vi "Werte ändern (DBL_0xZ.I._Rampen) (SubVI).vi"(0 "geladene Werte (Zeit (s); Wert)":dbl[][](array[numeric]), 1 "Zykluslänge":dbl, 3 "Info":string) -> (5 "Ausgang":dbl[][](array[numeric]) format="%.2f", 6 "Sperre":bool)   [LabVIEW 2010]
panel:
  out "abkühlen C°/s":dbl[](array[numeric])
  in  "abkühlen C°/s":dbl[](array[numeric])
  in  "Zykluslänge 2":dbl
  in  "abkühlen":dbl[](array[numeric])
  in  "Temp warm":dbl[](array[numeric])
  in  "°C/s":dbl[](array[numeric]) format="%#_1f"
  in  "Rampe los":dbl[](array[numeric])
  in  "Temp kalt":dbl[](array[numeric])
  out "abkühlen [s]":dbl[](array[numeric])
  out "Temp warm [°C ]":dbl[](array[numeric])
  out "°C/s":dbl[](array[numeric])
  out "Temp kalt [°C ]":dbl[](array[numeric])
  out "Rampe los [s]":dbl[](array[numeric])
  out "Fehlermeldung":string="Zeit ist größer als Zykluslänge"
  in  "löschen":bool
  out "XY Graph":cluster{"Array":dbl[], "Temp kalt":dbl[]}[](graph) caption="XY-Graph"
  out "Zykluslänge":dbl format="%.2f"
  out "Info":string
  in  "ändern":bool
  in  "Stopp":bool
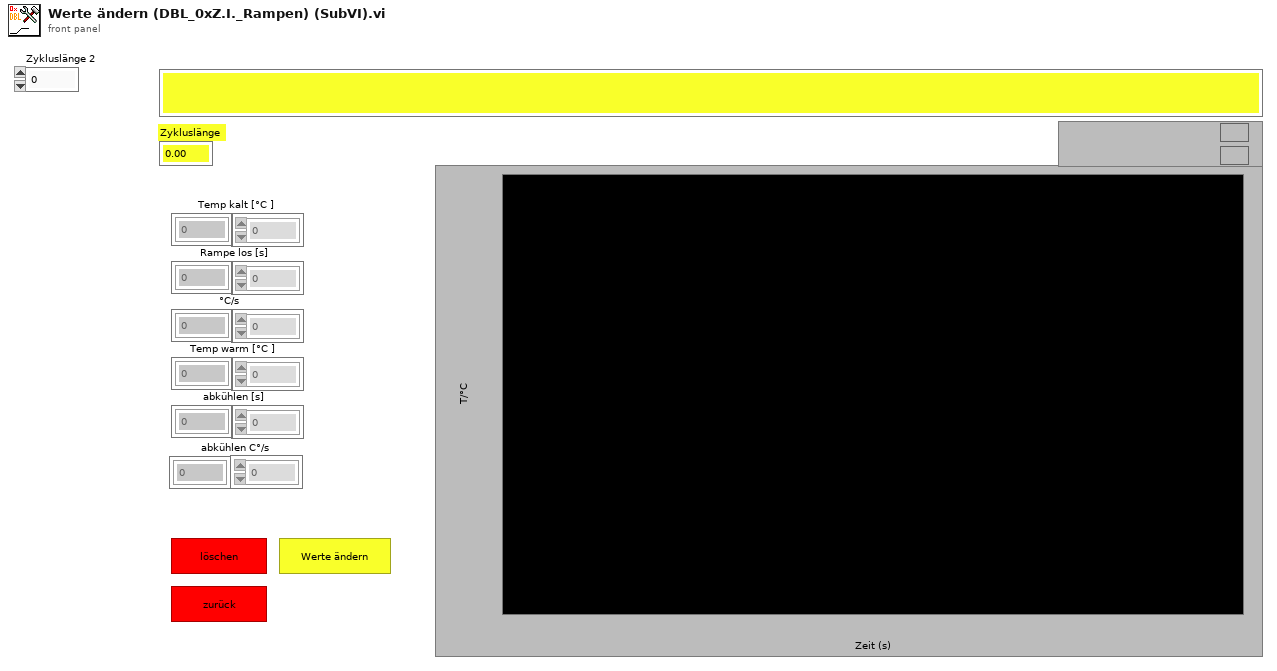
[diagram p1: front panel]
types:
  T1 = cluster{"Array":dbl[], "geladene Werte (Zeit (s); Wert)":dbl[]}
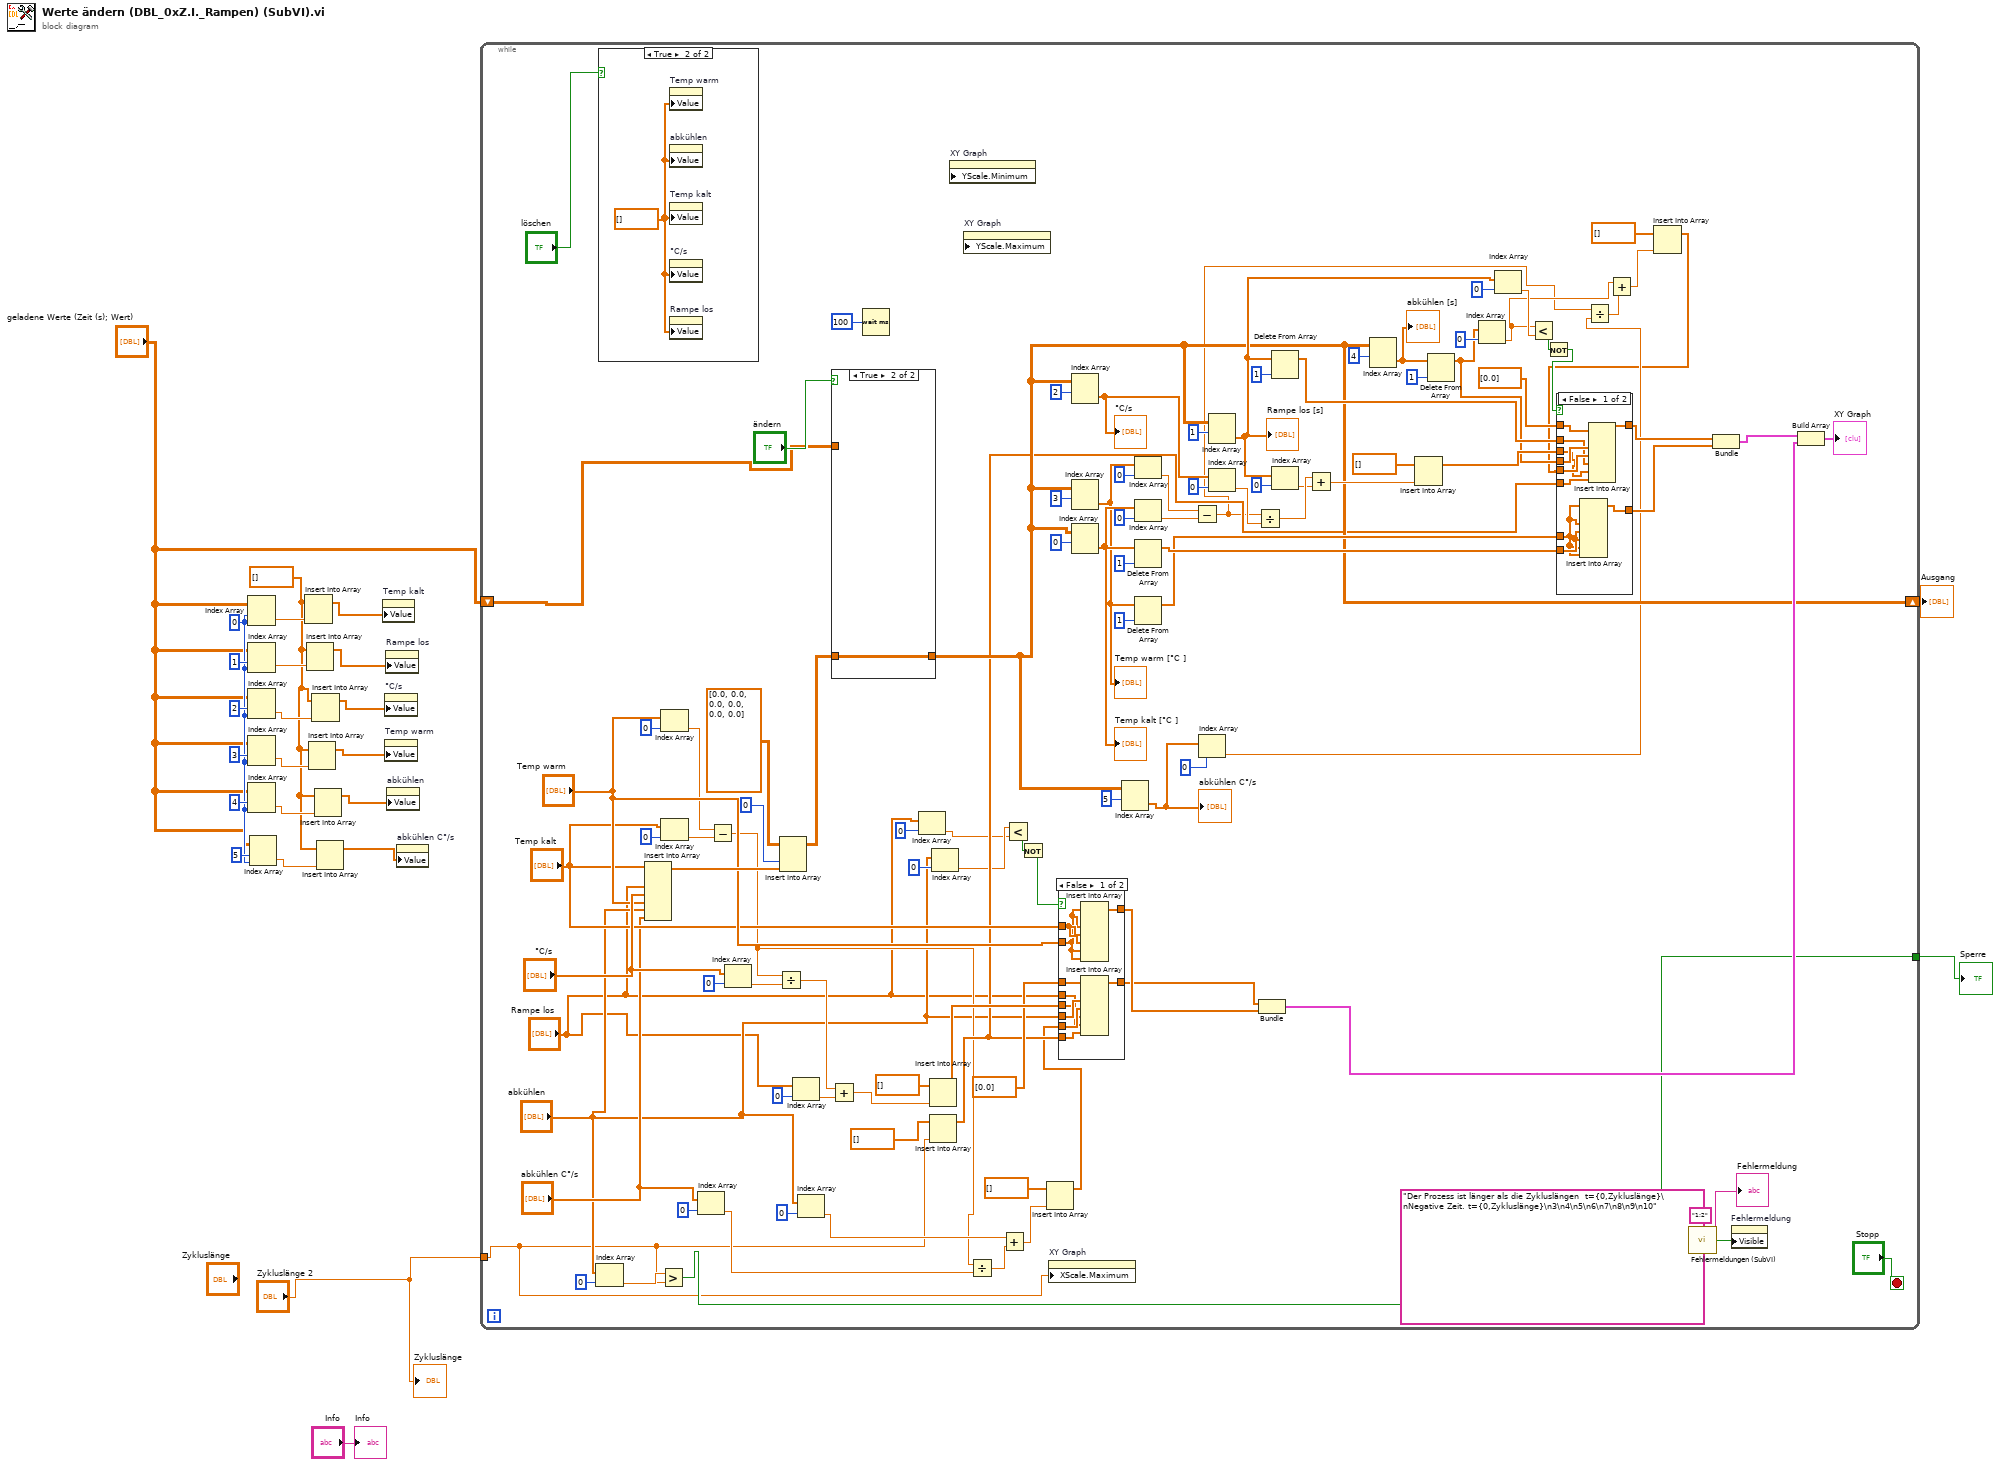
[diagram p0: block diagram]
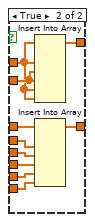
[diagram p2: hidden frame]
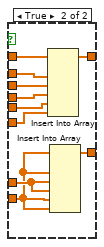
[diagram p3: hidden frame]
diagram:
  w2 = dbl[] [] ("Array")
  w4 = 0 ("Deaktivierter Index (Spalte)")
  n1 = Index Array(array="geladene Werte (Zeit (s); Wert)", index (row)=w4, index (col)=w4) -> (element=w18:dbl)
  n2 = Index Array(array="geladene Werte (Zeit (s); Wert)", index (row)=1 ("Deaktivierter Index (Zeile)"), index (col)=w4) -> (element=w17:dbl)
  n3 = Index Array(array="geladene Werte (Zeit (s); Wert)", index (row)=2 ("Deaktivierter Index (Zeile)"), index (col)=w4) -> (element=w16:dbl)
  n4 = Index Array(array="geladene Werte (Zeit (s); Wert)", index (row)=3 ("Deaktivierter Index (Zeile)"), index (col)=w4) -> (element=w15:dbl)
  n5 = Index Array(array="geladene Werte (Zeit (s); Wert)", index (row)=4 ("Deaktivierter Index (Zeile)"), index (col)=w4) -> (element=w14:dbl)
  n6 = Index Array(array="geladene Werte (Zeit (s); Wert)", index (row)=5 ("Deaktivierter Index (Zeile)"), index (col)=w4) -> (element=w5:dbl)
  n7 = Insert Into Array(array=w2, new element=w18) -> (w10:dbl[])  [unwired: 1 in]
  n8 = Insert Into Array(array=w2, new element=w17) -> (w13:dbl[])  [unwired: 1 in]
  n9 = Insert Into Array(array=w2, new element=w15) -> (w9:dbl[])  [unwired: 1 in]
  n10 = Insert Into Array(array=w2, new element=w16) -> (w12:dbl[])  [unwired: 1 in]
  n11 = Insert Into Array(array=w2, new element=w14) -> (w11:dbl[])  [unwired: 1 in]
  n12 = Insert Into Array(array=w2, new element=w5) -> (w1:dbl[])  [unwired: 1 in]
  n13 = property on="Temp kalt" class="Arr (strikt)"("Value"=w10) -> ()  [unwired: 2 in, 2 out]
  n14 = property on="°C/s" class="Arr (strikt)"("Value"=w12) -> ()  [unwired: 2 in, 2 out]
  n15 = property on="Temp warm" class="Arr (strikt)"("Value"=w9) -> ()  [unwired: 2 in, 2 out]
  n16 = property on="Rampe los" class="Arr (strikt)"("Value"=w13) -> ()  [unwired: 2 in, 2 out]
  n17 = property on="abkühlen" class="Arr (strikt)"("Value"=w11) -> ()  [unwired: 2 in, 2 out]
  n18 = property on="abkühlen C°/s" class="Arr (strikt)"("Value"=w1) -> ()  [unwired: 2 in, 2 out]
  n19 = while {
    shift-right: [w56] -> w24
    shift-left: "geladene Werte (Zeit (s); Wert)" -> [w73]
    tunnel: "Zykluslänge 2" -> [w25]
    tunnel: [w65] -> w8
    stop <- "Stopp" stop-if-true
    n20 = Index Array(array="abkühlen", index=0 ("Index")) -> (element=w71:dbl)
    n21 = case shown="True" "löschen" {
      frame False {
      }
      frame True {
        w173 = dbl[] [] ("neue Werte (Zeit (s); Wert)")
        n22 = property on="Temp warm" class="Arr (strikt)"("Value"=w173) -> ()  [unwired: 2 in, 2 out]
        n23 = property on="abkühlen" class="Arr (strikt)"("Value"=w173) -> ()  [unwired: 2 in, 2 out]
        n24 = property on="Temp kalt" class="Arr (strikt)"("Value"=w173) -> ()  [unwired: 2 in, 2 out]
        n25 = property on="°C/s" class="Arr (strikt)"("Value"=w173) -> ()  [unwired: 2 in, 2 out]
        n26 = property on="Rampe los" class="Arr (strikt)"("Value"=w173) -> ()  [unwired: 2 in, 2 out]
      }
    }
    n27 = Insert Into Array(array="Temp kalt", new element #1="Rampe los", new element #2="°C/s", new element #3="Temp warm", new element #4="abkühlen", new element #5="abkühlen C°/s") -> (w129:dbl[])  [unwired: 1 in]
    n28 = Greater?(x=w71, y=w25) -> (0:w70:bool)
    n29 = Index Array(array="Temp warm", index=0 ("Index")) -> (element=w106:dbl)
    n30 = Index Array(array="Temp kalt", index=0 ("Index")) -> (element=w104:dbl)
    n31 = Index Array(array="abkühlen C°/s", index=0 ("Index")) -> (element=w34:dbl)
    n32 = Subtract(x=w106, y=w104) -> (x-y=w37:dbl)
    n33 = Index Array(array="°C/s", index=0 ("Index")) -> (element=w105:dbl)
    n34 = Divide(x=w37, y=w105) -> (x/y=w120:dbl)
    n35 = Insert Into Array(array=dbl[][] [[0.0], [0.0], [0.0], [0.0], [0.0], [0.0]], index (col)=0 ("Deaktivierter Index (Spalte)"), new element=w129) -> (w126:dbl[][])  [unwired: 1 in]
    n36 = Index Array(array="Rampe los", index=0 ("Index")) -> (element=w103:dbl)
    n37 = Index Array(array="abkühlen", index=0 ("Index")) -> (element=w39:dbl)
    n38 = Add(x=w120, y=w103) -> (x+y=w118:dbl)
    n39 = case shown="True" "ändern" {
      tunnel: w73 -> [w174 _]
      tunnel: [w174 w175] -> w56
      tunnel: w126 -> [_ w175]
      frame False {
      }
      frame True {
      }
    }
    n40 = Wait (ms)(milliseconds to wait=u32 100 ("Zu wartende ms")) -> ()  [unwired: 1 out]
    n41 = Index Array(array="Rampe los", index=0 ("Index")) -> (element=w27:dbl)
    n42 = Insert Into Array(array=dbl[] [] ("Array"), new element=w118) -> (w117:dbl[])  [unwired: 1 in]
    n43 = Insert Into Array(array=dbl[] [] ("Array"), new element=w25) -> (w45:dbl[])  [unwired: 1 in]
    n44 = Index Array(array="abkühlen", index=0 ("Index")) -> (element=w28:dbl)
    n45 = property on="XY Graph" class="XYGraph (strikt)" props=["YScale", "Minimum"]() -> ()  [unwired: 3 in, 2 out]
    n46 = property on="XY Graph" class="XYGraph (strikt)" props=["YScale", "Maximum"]() -> ()  [unwired: 3 in, 2 out]
    n47 = Divide(x=w37, y=w34) -> (x/y=w44:dbl)
    n48 = Add(x=w39, y=w44) -> (x+y=w42:dbl)
    n49 = Less?(x=w28, y=w27) -> (x < y?=w32:bool)
    n50 = Not(x=w32) -> (.not. x?=w31:bool)
    n51 = Insert Into Array(array=dbl[] [] ("Array"), new element=w42) -> (w41:dbl[])  [unwired: 1 in]
    n52 = property on="XY Graph" class="XYGraph (strikt)"("XScale.Maximum"=w25) -> ()  [unwired: 2 in, 2 out]
    n53 = case shown="False" w31 {
      tunnel: w117 -> [w136 w152]
      tunnel: [w142 w151] -> w115
      tunnel: [w141 w150] -> w114
      tunnel: dbl[] [0.0] ("Array") -> [w140 w149]
      tunnel: "Rampe los" -> [w137 w148]
      tunnel: "Temp warm" -> [w133 w147]
      tunnel: "Temp kalt" -> [w134 w146]
      tunnel: w45 -> [w135 w145]
      tunnel: w41 -> [w138 w144]
      tunnel: "abkühlen" -> [w139 w143]
      frame False {
        n54 = Insert Into Array(array=w133, new element #1=w133, new element #2=w134, new element #3=w134, new element #4=w133, new element #5=w133) -> (w142:dbl[])  [unwired: 1 in]
        n55 = Insert Into Array(array=w140, new element #1=w139, new element #2=w138, new element #3=w137, new element #4=w136, new element #5=w135) -> (w141:dbl[])  [unwired: 1 in]
      }
      frame True {
        n56 = Insert Into Array(array=w146, new element #1=w146, new element #2=w147, new element #3=w147, new element #4=w146, new element #5=w146) -> (w151:dbl[])  [unwired: 1 in]
        n57 = Insert Into Array(array=w149, new element #1=w148, new element #2=w152, new element #3=w143, new element #4=w144, new element #5=w145) -> (w150:dbl[])  [unwired: 1 in]
      }
    }
    n58 = Index Array(array=w56, index (row)=2 ("Index (Zeile)")) -> (element=w88:dbl[])  [unwired: 1 in]
    "°C/s" <- w88
    n59 = Index Array(array=w56, index (row)=3 ("Index (Zeile)")) -> (element=w79:dbl[])  [unwired: 1 in]
    "Temp warm [°C ]" <- w79
    n60 = Index Array(array=w56, index (row)=0 ("Index (Zeile)")) -> (element=w84:dbl[])  [unwired: 1 in]
    "Temp kalt [°C ]" <- w84
    n61 = Index Array(array=w56, index (row)=5 ("Index (Zeile)")) -> (element=w51:dbl[])  [unwired: 1 in]
    "abkühlen C°/s" <- w51
    n62 = Index Array(array=w79, index=0 ("Index")) -> (element=w53:dbl)
    n63 = Index Array(array=w84, index=0 ("Index")) -> (element=w86:dbl)
    n64 = Delete From Array(array=w84, index=1 ("Index")) -> (array with subset deleted=w83:dbl[])  [unwired: 1 in, 1 out]
    n65 = Delete From Array(array=w79, index=1 ("Index")) -> (array with subset deleted=w78:dbl[])  [unwired: 1 in, 1 out]
    n66 = Subtract(x=w53, y=w86) -> (x-y=w38:dbl)
    n67 = Index Array(array=w51, index=0 ("Index")) -> (element=w50:dbl)
    n68 = Index Array(array=w56, index (row)=1 ("Index (Zeile)")) -> (element=w61:dbl[])  [unwired: 1 in]
    "Rampe los [s]" <- w61
    n69 = Index Array(array=w88, index=0 ("Index")) -> (element=w87:dbl)
    n70 = Divide(x=w38, y=w87) -> (x/y=w93:dbl)
    n71 = Bundle("Array"=w114, "Temp kalt"=w115) -> (w90:cluster{"Array":dbl[], "Temp kalt":dbl[]})  [unwired: 1 in]
    n72 = Delete From Array(array=w61, index=1 ("Index")) -> (array with subset deleted=w81:dbl[])  [unwired: 1 in, 1 out]
    n73 = Index Array(array=w61, index=0 ("Index")) -> (element=w74:dbl)
    n74 = Add(x=w93, y=w74) -> (x+y=w95:dbl)
    n75 = Index Array(array=w56, index (row)=4 ("Index (Zeile)")) -> (element=w76:dbl[])  [unwired: 1 in]
    "abkühlen [s]" <- w76
    n76 = Insert Into Array(array=dbl[] [] ("Array"), new element=w95) -> (w96:dbl[])  [unwired: 1 in]
    n77 = Delete From Array(array=w76, index=1 ("Index")) -> (array with subset deleted=w63:dbl[])  [unwired: 1 in, 1 out]
    n78 = Index Array(array=w63, index=0 ("Index")) -> (element=w55:dbl)
    n79 = Index Array(array=w61, index=0 ("Index")) -> (element=w60:dbl)
    n80 = Less?(x=w55, y=w60) -> (x < y?=w59:bool)
    n81 = Not(x=w59) -> (.not. x?=w58:bool)
    n82 = Divide(x=w38, y=w50) -> (x/y=w54:dbl)
    n83 = Add(x=w55, y=w54) -> (x+y=w48:dbl)
    n84 = Insert Into Array(array=dbl[] [] ("Array"), new element=w48) -> (w47:dbl[])  [unwired: 1 in]
    n85 = case shown="False" w58 {
      tunnel: dbl[] [0.0] ("Array") -> [w160 w172]
      tunnel: [w162 w171] -> w98
      tunnel: [w161 w170] -> w97
      tunnel: w96 -> [w156 w169]
      tunnel: w45 -> [w155 w165]
      tunnel: w83 -> [w154 w163]
      tunnel: w81 -> [w157 w168]
      tunnel: w78 -> [w153 w167]
      tunnel: w63 -> [w159 w166]
      tunnel: w47 -> [w158 w164]
      frame False {
        n86 = Insert Into Array(array=w153, new element #1=w153, new element #2=w154, new element #3=w154, new element #4=w153, new element #5=w153) -> (w161:dbl[])  [unwired: 1 in]
        n87 = Insert Into Array(array=w160, new element #1=w159, new element #2=w158, new element #3=w157, new element #4=w156, new element #5=w155) -> (w162:dbl[])  [unwired: 1 in]
      }
      frame True {
        n88 = Insert Into Array(array=w172, new element #1=w168, new element #2=w169, new element #3=w166, new element #4=w164, new element #5=w165) -> (w171:dbl[])  [unwired: 1 in]
        n89 = Insert Into Array(array=w163, new element #1=w163, new element #2=w167, new element #3=w167, new element #4=w163, new element #5=w163) -> (w170:dbl[])  [unwired: 1 in]
      }
    }
    n90 = call "Fehlermeldungen (SubVI).vi"("Fehler 1"=w70, "Fehlermeldungen Namen"="Der Prozess ist länger als die Zykluslängen  t={0,Zykluslänge}\nNegative Zeit. t={0,Zykluslänge}\n3\n4\n5\n6\n7\n8\n9\n10", "Kritischefehler Positionen"="1;2") -> ("Fehlermeldung Ausgang"=→"Fehlermeldung":string, "Fehler?"=w69:bool, "Sperre"=w65:bool)  [unwired: 22 in]
    n91 = Bundle("Array"=w98, "geladene Werte (Zeit (s); Wert)"=w97) -> (w91:T1)  [unwired: 1 in]
    n92 = property on="Fehlermeldung" class="Str"("Visible"=w69) -> ()  [unwired: 2 in, 2 out]
    n93 = Build Array(w91, w90) -> (→"XY Graph":cluster{"Array":dbl[], "Temp kalt":dbl[]}[])
  }
  "Ausgang" <- w24
  "Sperre" <- w8
  "Info" <- "Info"
  "Zykluslänge" <- "Zykluslänge 2"
